vi "Central_Controller_KAFB.vi"() -> ()   [LabVIEW 2019]
uses:
  <vilib>/Modbus/master/Modbus Master.lvclass
  <vilib>/Modbus/master/Create Master Instance (TCP).vi
panel:
  out "ALL Reactive Power":sgl[](array[numeric])
  out "ALL Frequency":sgl[](array[numeric])
  out "ALL Inverter Real Power":sgl[](array[numeric])
  out "ALL Inverter Reactive Power":sgl[](array[numeric])
  out "ALL Generator DC Voltage":sgl[](array[numeric])
  out "ALL Generator DC Current":sgl[](array[numeric])
  out "ALL Solar DC Voltage":sgl[](array[numeric])
  out "ALL Solar DC Current":sgl[](array[numeric])
  in  "DER List":string[](array[string])=["Capstone", "Aquion", "Tesla", "Load Bank", "Motor 1", "Simpliphi 1", "LG Chem", "Outback 1", "Outback 2", "Sunny Island", "ESS", "Fuel Cells", "Sparkplug", "Fronius", "Suny Boy", "Motor 2"]
  out "data":T1
  in  "File Name":string
  out "error out 3":errorcluster
  in  "Folder":path=path "C:/Users/administrator.STONEEDGEPOWER/Desktop/Data"
  out "ALL Status":u16[](array[numeric])
  out "SYS Current Time":dbl format="%.3f"
  out "SYS DER Index":i32
  out "ALL Control Method":string[](array[string])
  out "ALL Logged":bool[](array[boolean])
  out "ALL Through Variable":sgl[](array[numeric])
  out "ALL Across Variable":sgl[](array[numeric])
  out "ALL State of Charge":sgl[](array[numeric])
  out "ALL Real Power":sgl[](array[numeric])
  out "ALL Microgrid Voltage":sgl[](array[numeric])
  in  "Tab Control Main":enum32{"Dashboard", "Comms Control"}(tab)
  out "DER12 Solar Power":sgl format="%#.1f"
  out "DER12 Inverter Power":sgl format="%#.1f"
  out "DER11 Solar Power":sgl format="%#.1f"
  out "DER11 Inverter Power":sgl format="%#.1f"
  out "DER10 Solar Power":sgl format="%#.1f"
  out "DER10 Inverter Power":sgl format="%#.1f"
  out "DER9 Solar Power":sgl format="%#.1f"
  out "DER9 Inverter Power":sgl format="%#.1f"
  out "DER8 Solar Power":sgl format="%#.1f"
  out "DER8 Inverter Power":sgl format="%#.1f"
  out "DER7 Solar Power":sgl format="%#.1f"
  out "DER7 Inverter Power":sgl format="%#.1f"
  out "DER6 Solar Power":sgl format="%#.1f"
  out "DER6 Inverter Power":sgl format="%#.1f"
  out "DER5 Solar Power":sgl format="%#.1f"
  out "DER5 Inverter Power":sgl format="%#.1f"
  out "DER4 Solar Power":sgl format="%#.1f"
  out "DER1 Across Variable":sgl format="%#.1f"
  out "DER0 Across Variable":sgl format="%#.1f"
  out "DER12 Flow":i32(ring)
  out "DER12State of Charge Figure":sgl(slide) scale=0.0..100.0
  out "DER12 State of Charge":sgl format="%#.1f"
  out "DER12 Real Power":sgl format="%.1f"
  in  "DER12 Login Button":bool
  out "DER12 Logged":bool
  out "DER12 DC Voltage":sgl format="%#.1f"
  out "DER12 AC Line-Line Voltage":sgl=209.57935 format="%.1f"
  out "DER12 State":string
  in  "DER12 Control Window Button":bool
  in  "DER12 Detail Window Button":bool
  out "DER11 State of Charge":sgl format="%#.1f"
  out "DER11 Flow":i32(ring)
  in  "DER11 Detail Window Button":bool
  out "DER11 State of Charge Figure":sgl(slide) scale=0.0..100.0
  in  "DER11 Login Button":bool
  out "DER11 Across Variable":sgl format="%#.2f"
  out "DER11 logged":bool
  out "DER11 AC Line-Line Votlage":sgl format="%.1f"
  out "DER11 Real Power":sgl format="%.1f"
  out "DER11 State":string
  in  "DER11 Control Window Button":bool
  out "DER10 Flow":i32(ring)
  out "DER10 State of Charge Figure":sgl(slide) scale=0.0..100.0
  out "DER10 State of Charge":sgl format="%#.1f"
  out "DER10 Real Power":sgl format="%.1f"
  in  "DER10 Login Button":bool
  out "DER10 Logged":bool
  out "DER10 DC Voltage":sgl format="%#.1f"
  out "DER10 AC Line-Line Voltage":sgl=209.57935 format="%.1f"
  out "DER10 State":string
  in  "DER10 Control Window Button":bool
  in  "DER10 Detail Window Button":bool
  out "DER9 State of Charge":sgl format="%#.1f"
  out "DER9 Flow":i32(ring)
  in  "DER9 Detail Window Button":bool
  out "DER9 State of Charge Figure":sgl(slide) scale=0.0..100.0
  in  "DER9 Login Button":bool
  out "DER9 Across Variable":sgl format="%#.2f"
  out "DER9 logged":bool
  out "DER9 AC Line-Line Votlage":sgl format="%.1f"
  out "DER9 Real Power":sgl format="%.1f"
  out "DER9 State":string
  in  "DER9 Control Window Button":bool
  out "DER8 Flow":i32(ring)
  out "DER8 State of Charge Figure":sgl(slide) scale=0.0..100.0
  out "DER8 State of Charge":sgl format="%#.1f"
  out "DER8 Real Power":sgl format="%.1f"
  in  "DER8 Login Button":bool
  out "DER8 Logged":bool
  out "DER8 DC Voltage":sgl format="%#.1f"
  out "DER8 AC Line-Line Voltage":sgl=209.57935 format="%.1f"
  out "DER8 State":string
  in  "DER8 Control Window Button":bool
  in  "DER8 Detail Window Button":bool
  out "DER7 State of Charge":sgl format="%#.1f"
  out "DER5 State of Charge":sgl format="%#.1f"
  out "DER7 Flow":i32(ring)
  in  "DER7 Detail Window Button":bool
  out "DER7 State of Charge Figure":sgl(slide) scale=0.0..100.0
  in  "DER7 Login Button":bool
  out "DER7 Across Variable":sgl format="%#.2f"
  out "DER7 logged":bool
  out "DER7 AC Line-Line Votlage":sgl format="%.1f"
  out "DER7 Real Power":sgl format="%.1f"
  out "DER7 State":string
  in  "DER7 Control Window Button":bool
  out "DER6 Flow":i32(ring)
  out "DER6 State of Charge Figure":sgl(slide) scale=0.0..100.0
  out "DER6 State of Charge":sgl format="%#.1f"
  out "DER6 Real Power":sgl format="%.1f"
  in  "DER6 Login Button":bool
  out "DER6 Logged":bool
  out "DER6 DC Voltage":sgl format="%#.1f"
  out "DER6 AC Line-Line Voltage":sgl=209.57935 format="%.1f"
  out "DER6 State":string
  in  "DER6 Control Window Button":bool
  in  "DER6 Detail Window Button":bool
  out "DER0 State of Charge":sgl format="%.1f"
  out "DER0 State of Charge Figure":sgl(slide) scale=0.0..100.0
  out "DER5 Flow":i32(ring)
  out "DER4 Flow":i32(ring)
  out "DER3 Flow":i32(ring)
  out "DER1 Flow":i32(ring)
  out "DER0 Flow":i32(ring)
  in  "DER2 Detail Window Button":bool
  in  "DER5 Detail Window Button":bool
  out "DER4 State of Charge Figure":sgl(slide) scale=0.0..100.0
  out "DER4 State of Charge":sgl format="%#.1f"
  out "DER4 Real Power":sgl format="%.1f"
  in  "DER4 Login Button":bool
  out "DER4 Logged":bool
  out "DER4 DC Voltage":sgl format="%#.1f"
  out "DER4 AC Line-Line Voltage":sgl=209.57935 format="%.1f"
  out "DER4 State":string
  out "DER5 State of Charge Figure":sgl(slide) scale=0.0..100.0
  in  "DER0 Login Button":bool
  in  "DER2 Login Button":bool
  in  "DER1 Login Button":bool
  out "DER1 Real Power Indicator 1":sgl format="%.1f"
  out "DER1 Reactive Power":sgl format="%#.1f"
  out "DER1 AC Line-Line Voltage":sgl format="%.1f"
  out "DER0 Real Power":sgl format="%#.1f"
  out "DER0 AC Line-Line Voltage":sgl format="%#.1f"
  out "DER2 AC Line-Line Voltage":sgl format="%.1f"
  out "DER2 Real Power":sgl format="%.1f"
  out "DER0 Logged":bool
  out "DER1 Logged":bool
  out "DER2 Logged":bool
  in  "DER3 Login Button":bool
  out "DER3 Logged":bool
  out "DER3 Real Power":sgl format="%#.1f"
  out "DER3 AC Line-Line Votlage":sgl format="%#.1f"
  in  "DER5 Login Button":bool
  out "DER5 Across Variable":sgl format="%#.2f"
  out "DER5 logged":bool
  out "DER5 AC Line-Line Votlage":sgl format="%.1f"
  out "DER5 Real Power":sgl format="%.1f"
  out "DER0 State":string
  out "DER1 State":string
  out "DER2 State":string
  out "DER3 State":string
  out "DER5 State":string
  in  "DER0 Control Window Button":bool
  in  "DER0 Detail Window Button":bool
  in  "DER1 Detail Window Button":bool
  in  "DER1 Control Window Button":bool
  in  "DER2 Control Window Button":bool
  in  "DER3 Control Window Button":bool
  in  "DER5 Control Window Button":bool
  in  "DER4 Control Window Button":bool
  in  "DER4 Detail Window Button":bool
  out "DER2 Control Mode":string="Slave Mode Droops"
  out "DER1 Control Mode":string="Slave Mode Droops"
  out "DER2 Flow":i32(ring)
  out "DER0 Control Mode":string="Slave Mode Droops"
  out "DER1 Real Power Indicator 2":sgl format="%.1f"
  in  "DER3 Detail Window Button":bool
  out "DER1 Frequency":sgl format="%#.1f"
  out "DER4 Inverter Power":sgl format="%#.1f"
  in  "Container":enum32{"Page 1"}(tab)
  in  "DER Type":string[](array[string])=["Central", "Central", "Central", "Central", "Nanogrid", "Nanogrid", "Nanogrid", "Nanogrid", "Nanogrid", "Nanogrid", "Nanogrid", "Nanogrid", "Nanogrid", "DER13", "DER14", "DER15"]
  out "ALL Error Indicator":bool[](array[boolean])
  out "ALL DER Current Error":errorcluster[](array[cluster])
  out "ALL DER Final Error":errorcluster[](array[cluster])
  in  "IP Address List":string[](array[string])=["10.1.32.65", "10.1.32.32", "10.1.32.95", "10.1.32.97", "10.1.32.45", "10.1.32.67", "10.1.32.70", "10.1.32.100", "10.1.32.69", "10.1.32.38", "10.1.32.43", "10.1.32.75", "10.1.32.74", "10.0.1.192", "10.0.1.207", "10.0.1.196"]
  in  "DER Label Name":string[](array[string])=["DER0", "DER1", "DER2", "DER3", "DER4", "DER5", "DER6", "DER7", "DER8", "DER9", "DER10", "DER11", "DER12", "DER13", "DER14", "DER15"]
  out "SYS Iteration":i32
  in  "stop":bool
  out "SYS Status":string="Reading"
  out "SYS Case":i32
  in  "Read Array":bool[](array[boolean])=[TRUE, TRUE, TRUE, TRUE, TRUE, TRUE, TRUE, TRUE, TRUE, TRUE, TRUE, FALSE, TRUE]
  # "DER0: Heila XX, Sinamics, 10.0.8.XX\nDER1: Heila XX, Socomec, 10.0.8.XX\nDER2: Heila XX, Alencon, 10.0.8.XX\nDER3: Heila XX, Polar Power, 10.0.8.XX\nDER4: Heila XX, Nanogrid 1 \nDER5: Heila XX, Nanogrid 2\nDER6: Heila XX, Nanogrid 3\nDER7: Heila XX, Nanogrid 4 \nDER8: Heila XX, Nanogrid 5\nDER9: Heila XX, Nanogrid 6\nDER10: Heila XX, Nanogrid 7 \nDER11: Heila XX, Nanogrid 8\nDER12: Heila XX, Nanogrid 9"
  # "Nanogrid 5"
  # "Nanogrid 7"
  # "Nanogrid 3"
  # "Nanogrid 1"
  # "Nanogrid 9"
  # "House"
  # "DETL"
  # "House"
  # "House"
  # "House"
  # "Battery"
  # "Generators"
  # "Status:"
  # "Status:"
  # "Status:"
  # "Status:"
  # "Status:"
  # "Sinamics + Energport"
  # "EPIC + Polar Power"
  # "V"
  # "V"
  # "V"
  # "V"
  # "V"
  # "Status:"
  # "Status:"
  # "Mode:"
  # "KAFB Microgrid in Real Time"
  # "V"
  # "SoC"
  # "%"
  # "SoC"
  # "%"
  # "SoC"
  # "%"
  # "SoC"
  # "%"
  # "SoC"
  # "%"
  # "Load:"
  # "Load:"
  # "Load:"
  # "Load:"
  # "Load:"
  # "Solar:"
  # "Solar:"
  # "Solar:"
  # "Solar:"
  # "Solar:"
  # "SoC"
  # "%"
  # "Inverter"
  # "Utility Grid"
  # "kW"
  # "kW"
  # "kW"
  # "kW"
  # "kW"
  # "kW"
  # "kW"
  # "kW"
  # "Socomec"
  # "V"
  # "V"
  # "V"
  # "V"
  # "V"
  # "V"
  # "V"
  # "V"
  # "Status:"
  # "Mode:"
  # "V ="
  # "V"
  # "f ="
  # "Hz"
  # "P ="
  # "kW"
  # "kW"
  # "kW"
  # "kW"
  # "kW"
  # "kW"
  # "kVAr"
  # "Q ="
  # "V"
  # "V"
  # "V"
  # "V"
  # "V"
  # "Solar"
  # "Nanogrid 8"
  # "Nanogrid 6"
  # "Nanogrid 4"
  # "Nanogrid 2"
  # "Laundry"
  # "House"
  # "House"
  # "PV + Alencon"
  # "House"
  # "Status:"
  # "Status:"
  # "Status:"
  # "Status:"
  # "Status:"
  # "Mode:"
  # "V"
  # "V"
  # "V"
  # "V"
  # "SoC"
  # "%"
  # "SoC"
  # "%"
  # "SoC"
  # "%"
  # "SoC"
  # "%"
  # "Load:"
  # "Load:"
  # "Load:"
  # "Load:"
  # "Solar:"
  # "Solar:"
  # "Solar:"
  # "Solar:"
  # "Program"
  # "Controllable DERs"
  # "DER0: Heila XX, Sinamics, 10.1.32.65\nDER1: Heila XX, Socomec, 10.1.32.32\nDER2: Heila XX, Alencon, 10.1.32.95\nDER3: Heila XX, Polar Power, 10.1.32.97\nDER4: Heila XX, Nanogrid 1, 10.1.32.45 \nDER5: Heila XX, Nanogrid 2, 10.1.32.67\nDER6: Heila XX, Nanogrid 3, 10.1.32.70\nDER7: Heila XX, Nanogrid 4, 10.1.32.100\nDER8: Heila XX, Nanogrid 5, 10.1.32.68\nDER9: Heila XX, Nanogrid 6, 10.1.32.38\nDER10: Heila XX, Nanogrid 7, 10.1.32.43\nDER11: Heila XX, Nanogrid 8\nDER12: Heila XX, Nanogrid 9"
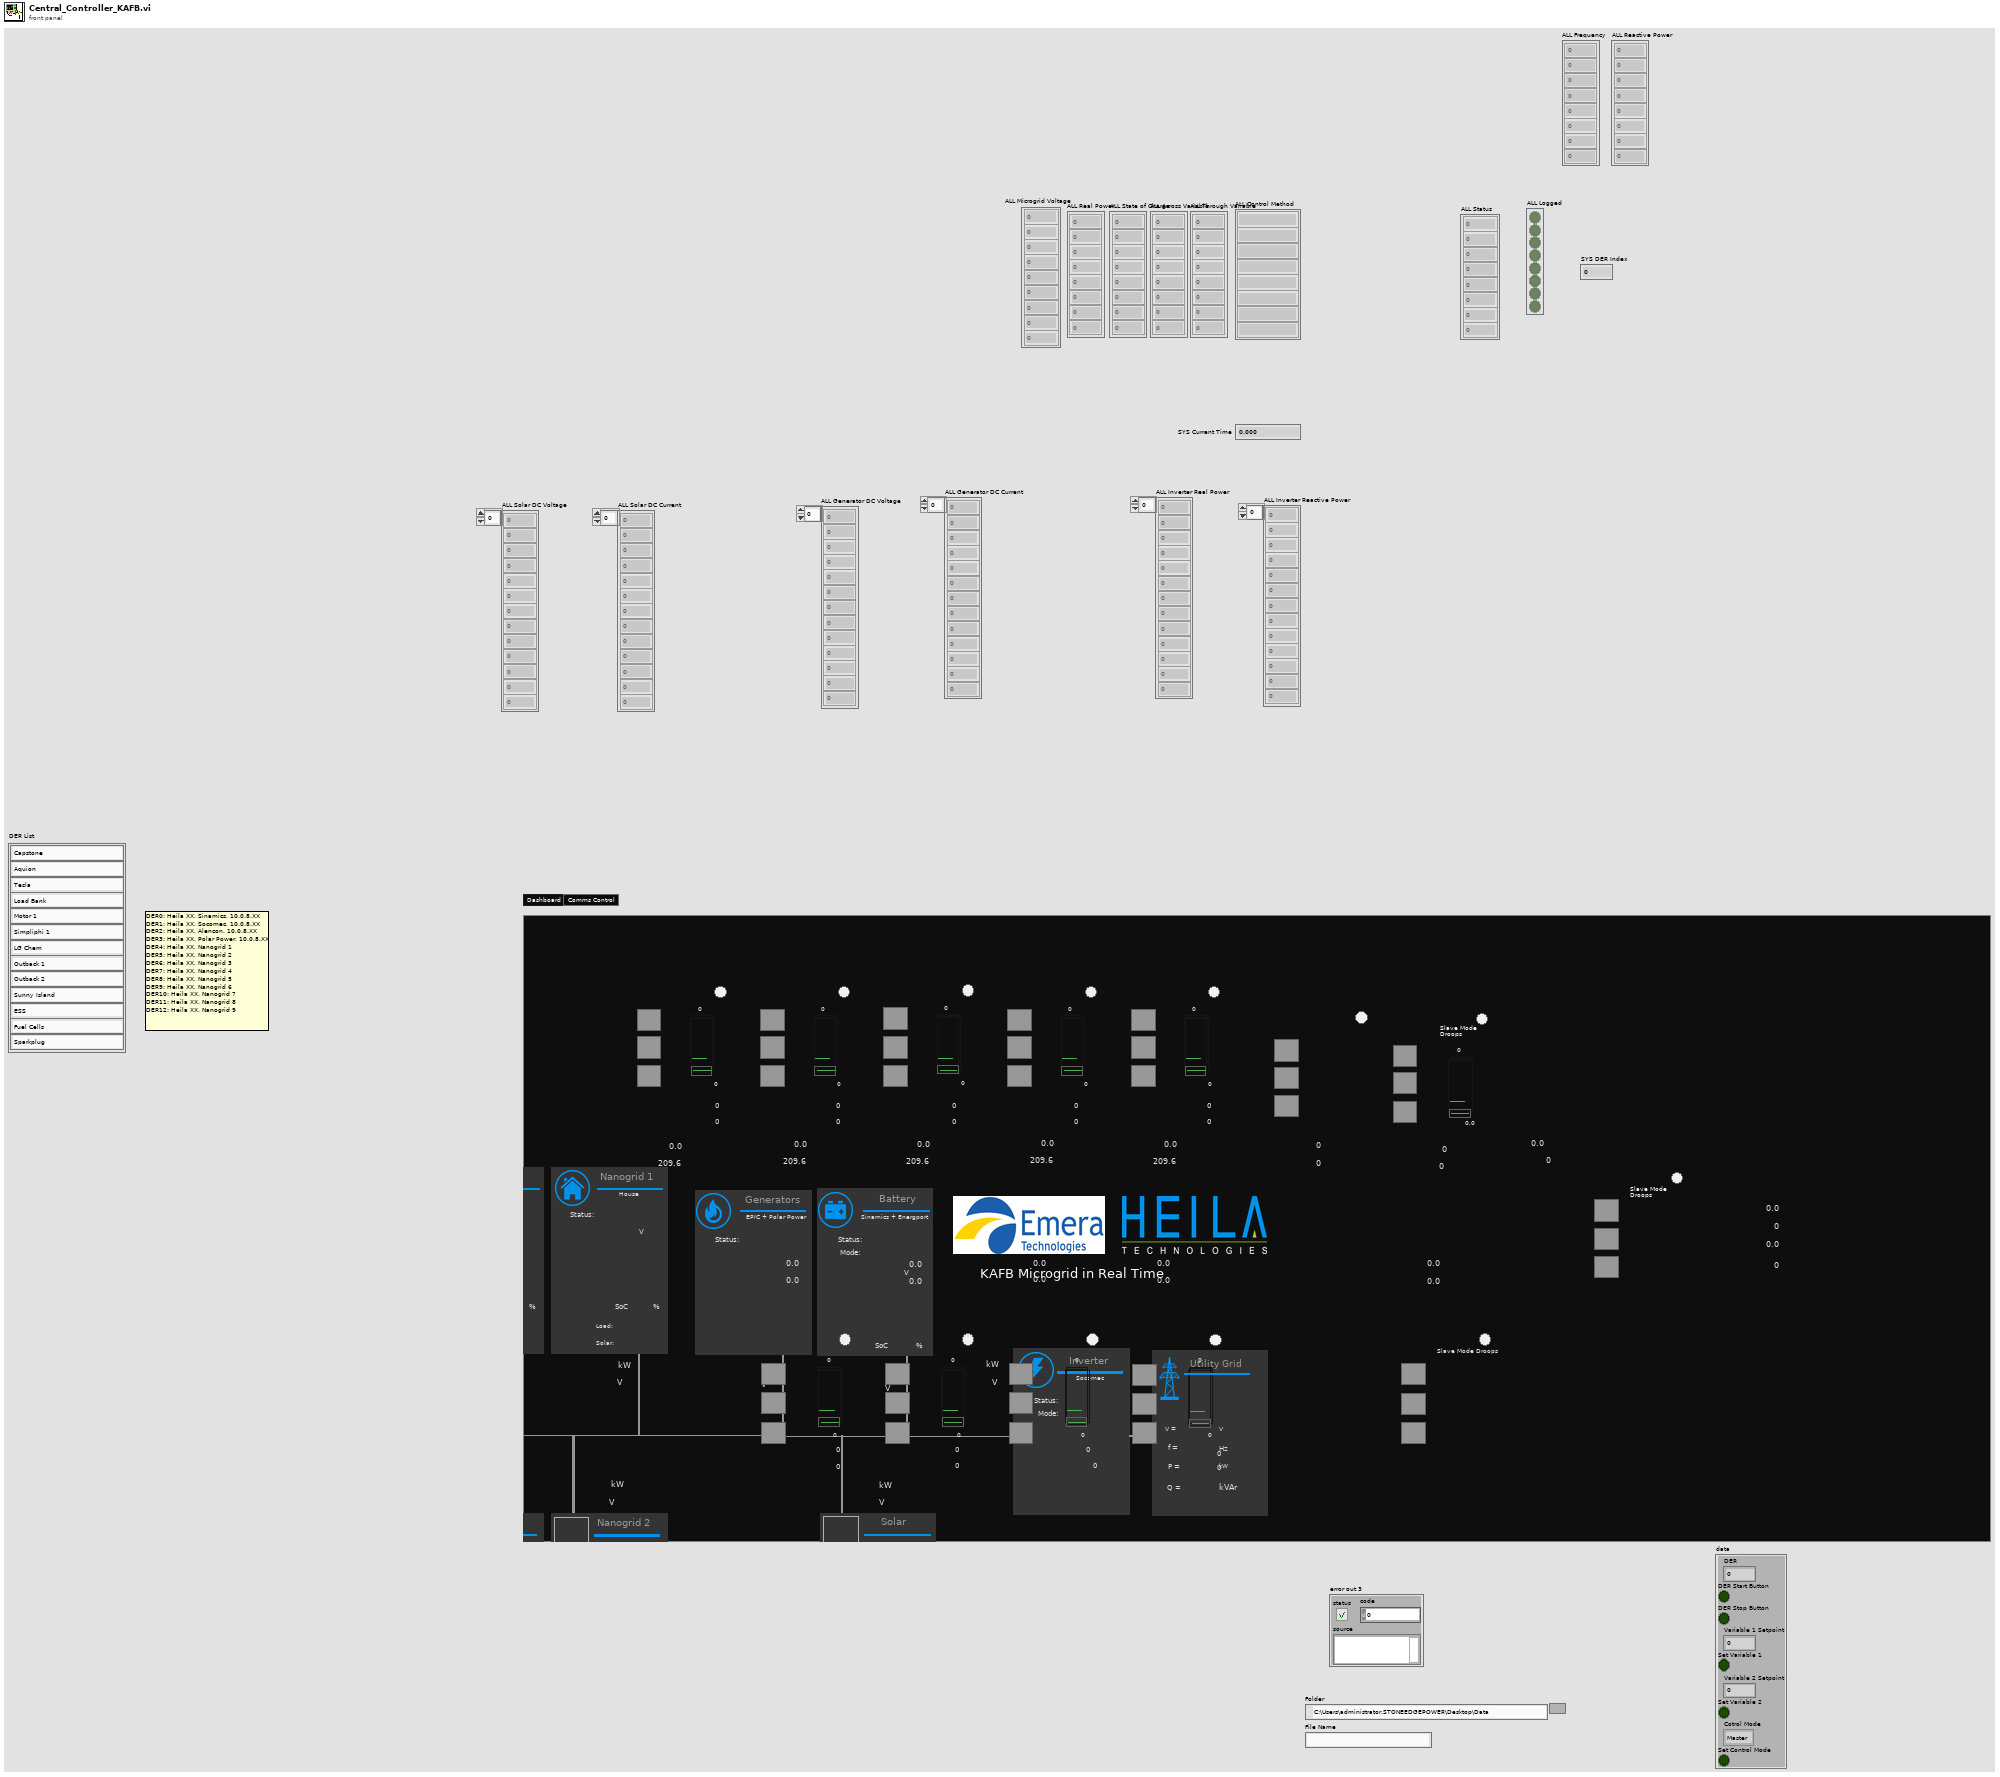
[diagram p1: front panel]
types:
  T1 = cluster{"DER":i32, "DER Start Button":bool, "DER Stop Button":bool, "Variable 1 Setpoint":sgl, "Set Variable 1":bool, "Variable 2 Setpoint":sgl, "Set Variable 2":bool, "Cotrol Mode":enum16{"Master", "Slave"}, "Set Control Mode":bool}
  T2 = enum16{"open", "replace", "create", "open or create", "replace or create", "replace or create with confirmation"}
  T3 = cluster{"Modbus master out":refnum<class "Modbus Master.lvclass">, "error out":errorcluster}[]
  T4 = enum32{"Invalid", "Standard", "Closed", "Hidden", "Minimized", "Maximized"}
  T5 = cluster{"Modbus master out":refnum<class "Modbus Master.lvclass">, "error out":errorcluster}
  T6 = enum32{"Bad", "Idle", "Run top level", "Running"}
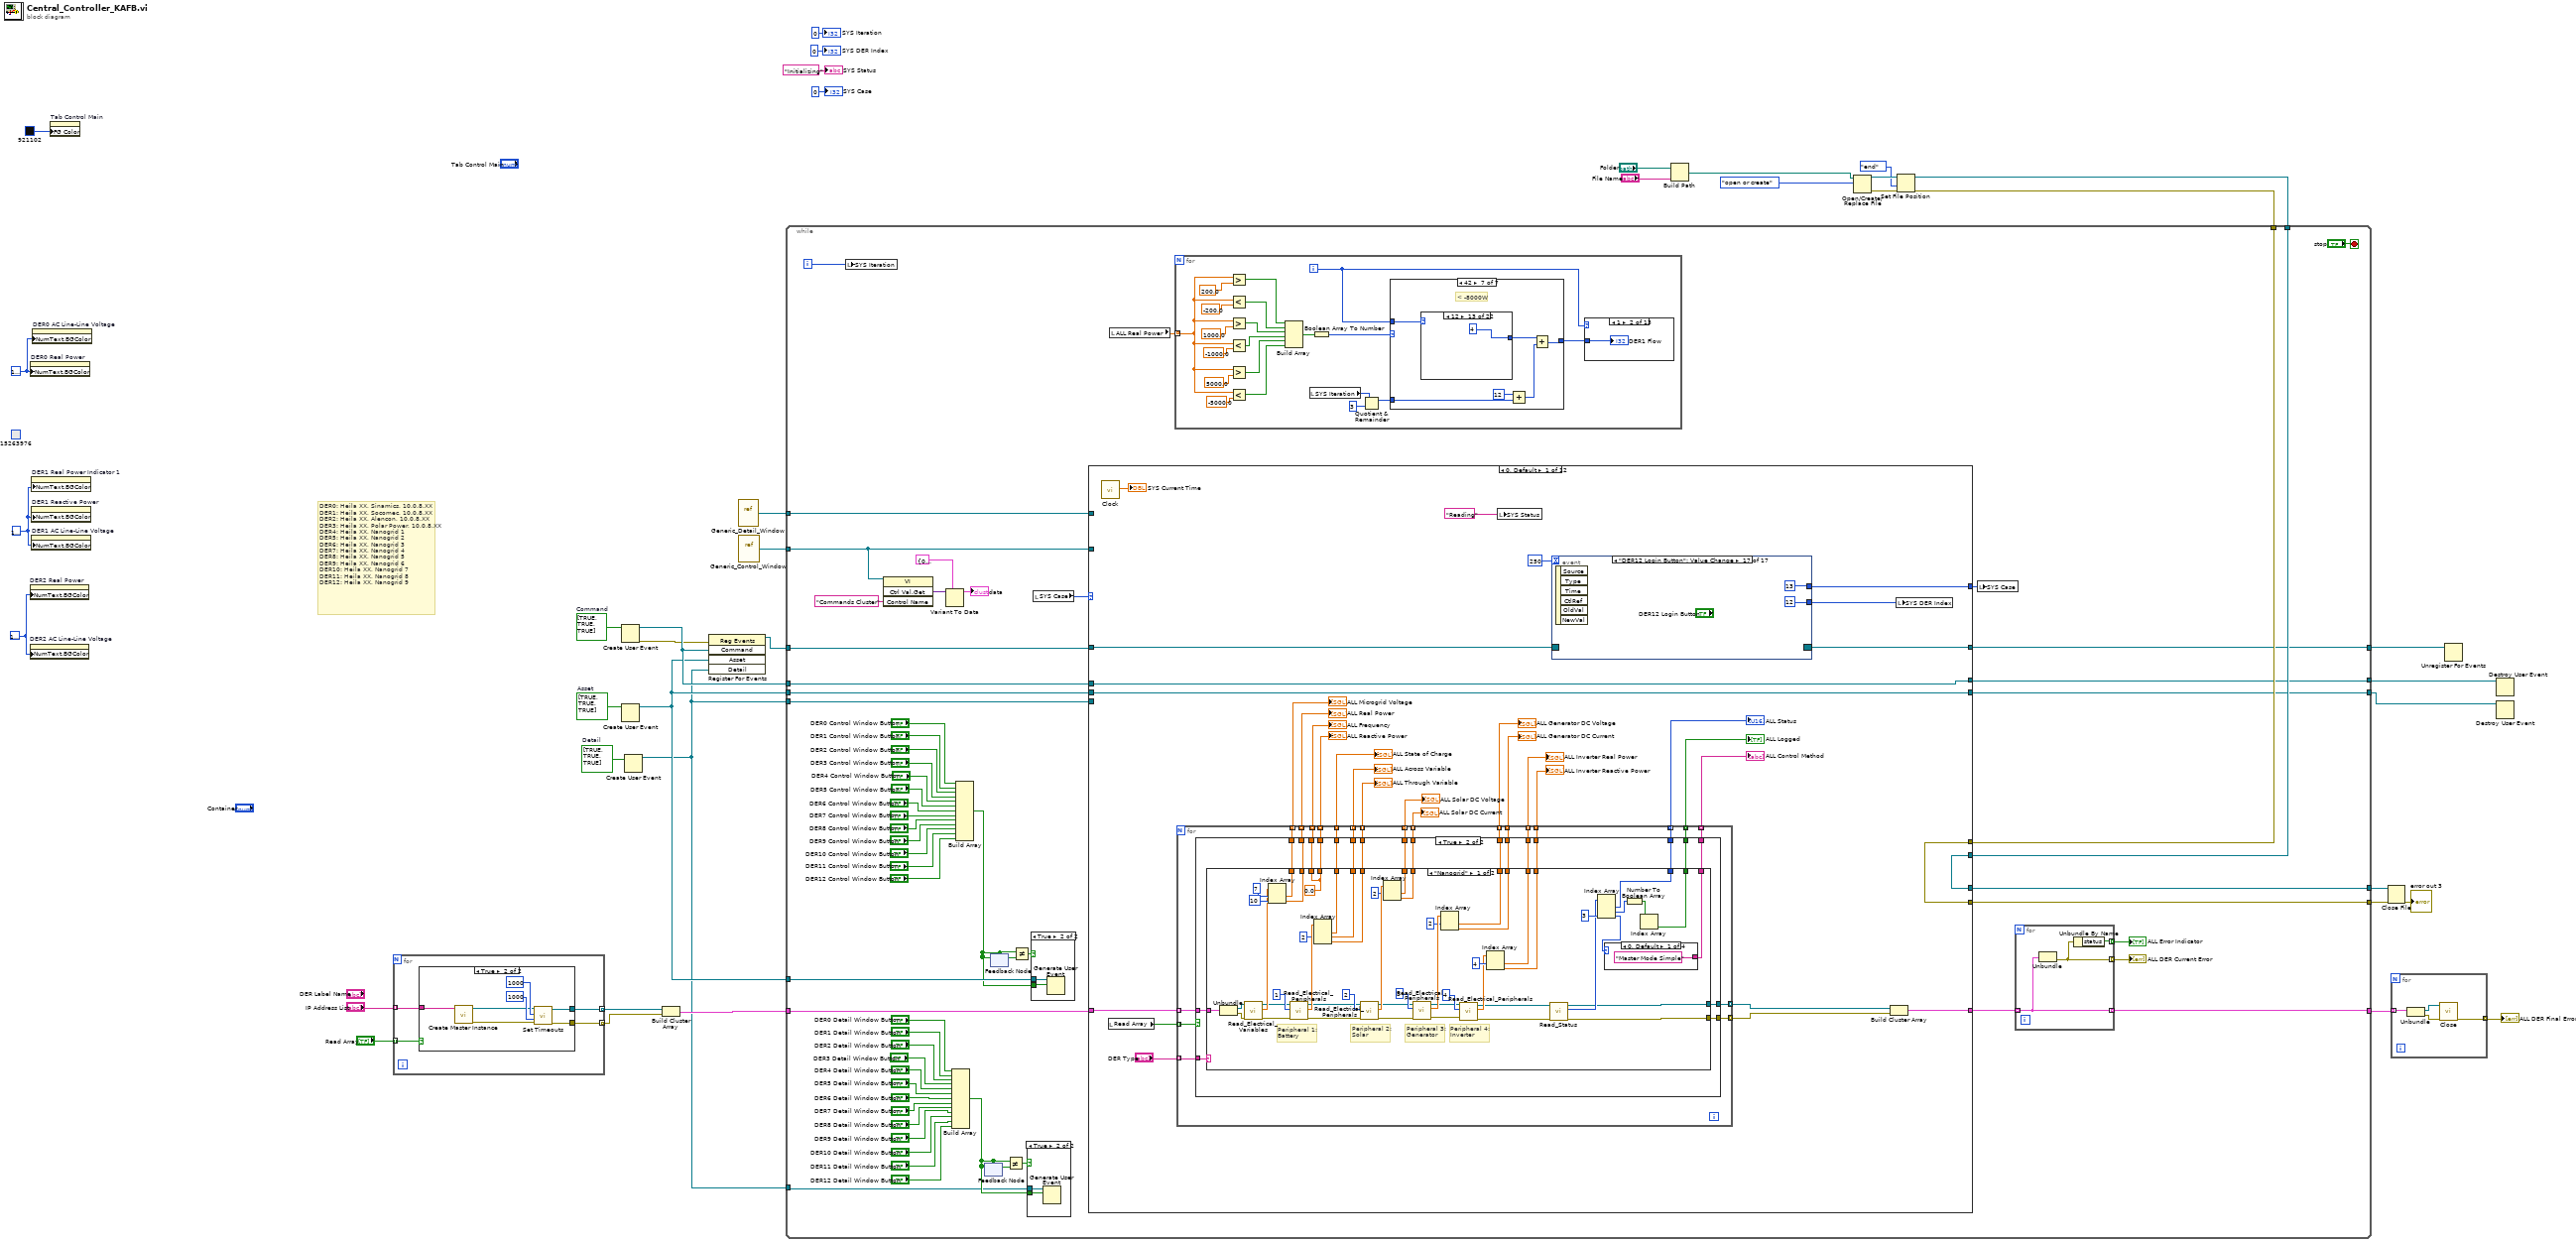
[diagram p0: block diagram]
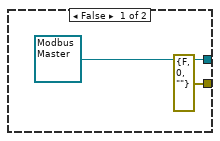
[diagram p2: hidden frame]
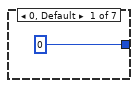
[diagram p5: hidden frame]
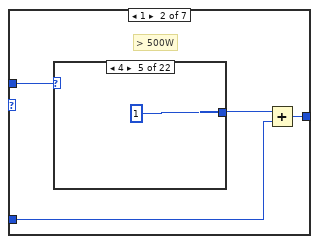
[diagram p6: hidden frame]
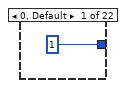
[diagram p7: hidden frame]
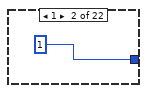
[diagram p8: hidden frame]
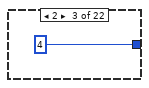
[diagram p9: hidden frame]
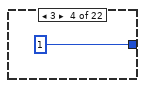
[diagram p10: hidden frame]
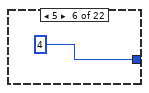
[diagram p11: hidden frame]
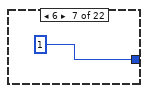
[diagram p12: hidden frame]
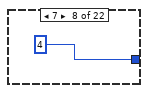
[diagram p13: hidden frame]
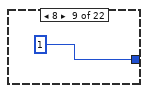
[diagram p14: hidden frame]
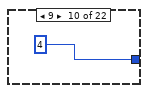
[diagram p15: hidden frame]
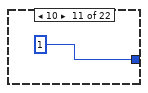
[diagram p16: hidden frame]
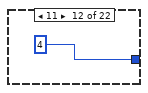
[diagram p17: hidden frame]
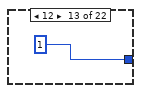
[diagram p18: hidden frame]
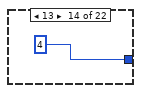
[diagram p19: hidden frame]
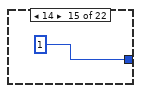
[diagram p20: hidden frame]
diagram:
  w4 = bool[] [TRUE, TRUE, TRUE]  # Detail
  w10 = bool[] [TRUE, TRUE, TRUE]  # Asset
  w13 = bool[] [TRUE, TRUE, TRUE]  # Command
  w36 = u32 16777216
  w37 = u32 16777216
  w38 = u32 16777216
  (unwired) u32 15263976
  # "DER0: Heila XX, Sinamics, 10.0.8.XX\nDER1: Heila XX, Socomec, 10.0.8.XX\nDER2: Heila XX, Alencon, 10.0.8.XX\nDER3: Heila XX, Polar Power, 10.0.8.XX\nDER4: Heila XX, Nanogrid 1 \nDER5: Heila XX, Nanogrid 2\nDER6: Heila XX, Nanogrid 3\nDER7: Heila XX, Nanogrid 4 \nDER8: Heila XX, Nanogrid 5\nDER9: Heila XX, Nanogrid 6\nDER10: Heila XX, Nanogrid 7 \nDER11: Heila XX, Nanogrid 8\nDER12: Heila XX, Nanogrid 9"
  n1 = property on="DER2 Real Power" class="DigNum (strict)"("NumText.BGColor"=w36) -> ()  [unwired: 2 in, 2 out]
  n2 = property on="DER2 AC Line-Line Voltage" class="DigNum (strict)"("NumText.BGColor"=w36) -> ()  [unwired: 2 in, 2 out]
  n3 = property on="DER0 Real Power" class="DigNum (strict)"("NumText.BGColor"=w38) -> ()  [unwired: 2 in, 2 out]
  n4 = property on="DER1 Real Power Indicator 1" class="DigNum (strict)"("NumText.BGColor"=w37) -> ()  [unwired: 2 in, 2 out]
  n5 = property on="DER1 Reactive Power" class="DigNum (strict)"("NumText.BGColor"=w37) -> ()  [unwired: 2 in, 2 out]
  n6 = property on="DER1 AC Line-Line Voltage" class="DigNum (strict)"("NumText.BGColor"=w37) -> ()  [unwired: 2 in, 2 out]
  n7 = property on="DER0 AC Line-Line Voltage" class="DigNum (strict)"("NumText.BGColor"=w38) -> ()  [unwired: 2 in, 2 out]
  n8 = property on="Tab Control Main" class="TabCtl (strict)"("FG Color"=u32 921102) -> ()  [unwired: 2 in, 2 out]
  n9 = for {
    tunnel: "IP Address List" -> [w44] mode=indexing
    tunnel: [w43] -> w35 mode=indexing
    tunnel: [w42] -> w34 mode=indexing
    tunnel: "Read Array" -> [w41] mode=indexing
    n10 = case shown="True" w41 {
      tunnel: w44 -> [_ w53]
      tunnel: [refnum<class "Modbus Master.lvclass"> refnum ("Modbus master out") w50] -> w43
      tunnel: [errorcluster {"status"=FALSE, "code"=0, "source"=""} ("error out") w49] -> w42
      frame False {
      }
      frame True {
        n11 = call-poly <vilib>:"Create Master Instance.vi"("address"=w53) -> ("error out"=w47:errorcluster, "TCP master instance"=w48:refnum<class "Modbus Master.lvclass">)  [unwired: 9 in]
        n12 = call <vilib>:"Set Timeouts.vi"("error in (no error)"=w47, "write operation timeout (ms)"=1000 ("Write Timeout"), "read operation timeout (ms)"=1000 ("Read Timeout"), "Modbus master in"=w48) -> ("error out"=w49:errorcluster, "Modbus master out"=w50:refnum<class "Modbus Master.lvclass">)  [unwired: 6 in]
      }
    }
  }
  n13 = Create User Event(user event datatype=w13) -> (user event=w11:refnum<user-event>, error out=w7:errorcluster)  [unwired: 1 in]
  n14 = Create User Event(user event datatype=w10) -> (user event=w6:refnum<user-event>)  [unwired: 1 in, 1 out]
  n15 = Create User Event(user event datatype=w4) -> (user event=w2:refnum<user-event>)  [unwired: 1 in, 1 out]
  n16 = Build Cluster Array(w35, w34) -> (w33:T3)
  n17 = register-events(error in=w7, w11, w6, w2) -> (reference out=w12:refnum<event-registration>)  [unwired: 1 in, 1 out]
  n18 = vi-ref "Generic_Detail_Window.vi"() -> (w3:refnum<vi>)
  n19 = vi-ref "Generic_Control_Window.vi"() -> (w14:refnum<vi>)
  n20 = Build Path(base path="Folder", name or relative path="File Name") -> (appended path=w15:path)
  n21 = Open/Create/Replace File(file path (use dialog)=w15, operation (0:open)=T2."open or create") -> (refnum out=w25:refnum<file>, error out=w24:errorcluster)  [unwired: 4 in, 1 out]
  n22 = Set File Position(refnum=w25, from (0:start)=enum16{"start", "end", "current"}."end", error in=w24) -> (refnum out=w19:refnum<file>, error out=w18:errorcluster)  [unwired: 1 in]
  n23 = while {
    tunnel: w33 -> [w112]
    tunnel: [w108] -> w27
    tunnel: [w106] -> w22
    tunnel: [w105] -> w21
    tunnel: w19 -> [w104]
    tunnel: w18 -> [w103]
    tunnel: w14 -> [w83]
    tunnel: w11 -> [w101]
    tunnel: w6 -> [w92]
    tunnel: [w89] -> w8
    tunnel: w6 -> [w88]
    tunnel: [w87] -> w5
    tunnel: w12 -> [w102]
    tunnel: [w90] -> w9
    tunnel: w2 -> [w74]
    tunnel: w3 -> [w73]
    tunnel: w2 -> [w72]
    i -> [w55]
    stop <- "stop" stop-if-true
    n24 = local write "SYS Iteration"(w55) -> ()
    n25 = invoke class="VI" method="Ctrl Val.Get"(reference=w83, "Control Name"="Commands Cluster") -> ("Get Control Value Variant"=w100:variant)  [unwired: 2 in, 3 out]
    n26 = Variant To Data(type=T1 {"DER"=0, "DER Start Button"=FALSE, "DER Stop Button"=FALSE, "Variable 1 Setpoint"=0.0, "Set Variable 1"=FALSE, "Variable 2 Setpoint"=0.0, "Set Variable 2"=FALSE, "Cotrol Mode"=enum."Slave", "Set Control Mode"=FALSE} ("Commands Cluster 2"), Variant=w100) -> (data=→"data":T1)  [unwired: 1 in, 1 out]
    n27 = Build Array("DER0 Detail Window Button", "DER1 Detail Window Button", "DER2 Detail Window Button", "DER3 Detail Window Button", "DER4 Detail Window Button", "DER5 Detail Window Button", "DER6 Detail Window Button", "DER7 Detail Window Button", "DER8 Detail Window Button", "DER9 Detail Window Button", "DER10 Detail Window Button", "DER11 Detail Window Button", "DER12 Detail Window Button") -> (w76:bool[])
    n28 = Build Array("DER0 Control Window Button", "DER1 Control Window Button", "DER2 Control Window Button", "DER3 Control Window Button", "DER4 Control Window Button", "DER5 Control Window Button", "DER6 Control Window Button", "DER7 Control Window Button", "DER8 Control Window Button", "DER9 Control Window Button", "DER10 Control Window Button", "DER11 Control Window Button", "DER12 Control Window Button") -> (w91:bool[])
    n29 = feedback #1(w76) -> (w77:bool[])
    n30 = feedback-in #1(w76) -> ()
    n31 = feedback-in #2(w91) -> ()
    n32 = feedback #2(w91) -> (w93:bool[])
    n33 = Not Equal?(x=w76, y=w77) -> (x != y?=w75:bool)
    n34 = Not Equal?(x=w91, y=w93) -> (x != y?=w86:bool)
    n35 = case shown="True" w75 {
      tunnel: w74 -> [_ w116]
      tunnel: w76 -> [_ w115]
      frame False {
      }
      frame True {
        n36 = Generate User Event(user event=w116, event data cluster=w115) -> ()  [unwired: 2 in, 2 out]
      }
    }
    n37 = case shown="True" w86 {
      tunnel: w92 -> [_ w118]
      tunnel: w91 -> [_ w117]
      frame False {
      }
      frame True {
        n38 = Generate User Event(user event=w118, event data cluster=w117) -> ()  [unwired: 2 in, 2 out]
      }
    }
    n39 = local read "SYS Case"() -> (w113:i32)
    n40 = case shown="0, Default" w113 {
      tunnel: [w351 2 0 0 0 0 0 0 0 0 w877 w907] -> w82
      tunnel: [w346 w568 w742 w747 w761 w778 w811 w824 w842 w861 w881 w909] -> w111
      tunnel: w112 -> [w349 w568 w742 w749 w762 w782 w812 w823 w843 w862 w881 w909]
      tunnel: [w336 _ w739 _ _ _ _ _ _ _ _ _] -> w106
      tunnel: [w337 _ w738 _ _ _ _ _ _ _ _ _] -> w105
      tunnel: w104 -> [w336 _ w737 _ _ _ _ _ _ _ _ _]
      tunnel: w103 -> [w337 _ w736 _ _ _ _ _ _ _ _ _]
      tunnel: w83 -> [_ _ _ _ _ _ _ _ _ _ w878 _]
      tunnel: w102 -> [w335 w559 w732 _ _ _ _ _ _ _ _ _]
      tunnel: [w334 w559 w732 _ _ _ _ _ _ _ _ _] -> w90
      tunnel: w101 -> [w333 _ _ _ _ _ _ _ _ _ w880 _]
      tunnel: [w333 _ _ _ _ _ _ _ _ _ _ _] -> w89
      tunnel: w88 -> [w332 _ _ _ _ _ _ _ _ _ _ _]
      tunnel: [w332 _ _ _ _ _ _ _ _ _ _ _] -> w87
      tunnel: w73 -> [_ _ _ _ _ _ _ _ _ _ _ w906]
      tunnel: w72 -> [_ _ _ _ _ _ _ _ _ _ _ _]
      frame 0, Default {
        n41 = call "Clock.vi"() -> ("SYS Current Time"=→"SYS Current Time":dbl)  [unwired: 11 in]
        n42 = local read "Read Array"() -> (w330:bool[])
        n43 = for {
          tunnel: w349 -> [w373] mode=indexing
          tunnel: [w372] -> w348 mode=indexing
          tunnel: [w371] -> w347 mode=indexing
          tunnel: [w364] -> w345 mode=indexing
          tunnel: [w370] -> w344 mode=indexing
          tunnel: [w367] -> w343 mode=indexing
          tunnel: [w366] -> w342 mode=indexing
          tunnel: [w369] -> w340 mode=indexing
          tunnel: [w368] -> w341 mode=indexing
          tunnel: [w365] -> w338 mode=indexing
          tunnel: w330 -> [w363] mode=indexing
          tunnel: "DER Type" -> [w362] mode=indexing
          tunnel: [w361] -> w328 mode=indexing
          tunnel: [w360] -> w326 mode=indexing
          tunnel: [w359] -> w327 mode=indexing
          tunnel: [w358] -> w325 mode=indexing
          tunnel: [w357] -> w324 mode=indexing
          tunnel: [w356] -> w323 mode=indexing
          tunnel: [w355] -> w322 mode=indexing
          tunnel: [w354] -> w321 mode=indexing
          tunnel: [w353] -> w320 mode=indexing
          n44 = case shown="True" w363 {
            tunnel: w373 -> [w377 w400]
            tunnel: [w376 w399] -> w372
            tunnel: [w375 w398] -> w371
            tunnel: [w374 w391] -> w370
            tunnel: ["OFF" w397] -> w369
            tunnel: [FALSE w396] -> w368
            tunnel: [w374 w390] -> w367
            tunnel: [w374 w389] -> w366
            tunnel: [u16 1 ("register") w395] -> w365
            tunnel: [w374 w392] -> w364
            tunnel: w362 -> [_ w394]
            tunnel: [w374 w393] -> w361
            tunnel: [w374 w388] -> w360
            tunnel: [w374 w387] -> w359
            tunnel: [w374 w386] -> w358
            tunnel: [w374 w385] -> w357
            tunnel: [w374 w384] -> w356
            tunnel: [w374 w383] -> w355
            tunnel: [w374 w382] -> w354
            tunnel: [w374 w381] -> w353
            frame False {
              w374 = sgl 0.0
              n45 = Unbundle(w377) -> ("Modbus master out"=w376:refnum<class "Modbus Master.lvclass">, "error out"=w375:errorcluster)
            }
            frame True {
              n46 = case shown="\"Nanogrid\"" w394 {
                tunnel: w400 -> [w448 w486]
                tunnel: [w436 w483] -> w399
                tunnel: [w435 w482] -> w398
                tunnel: [w433 w475] -> w397
                tunnel: [w434 w473] -> w396
                tunnel: [w432 w472] -> w395
                tunnel: [w431 w468] -> w393
                tunnel: [w430 w466] -> w392
                tunnel: [w427 w458] -> w391
                tunnel: [w426 w464] -> w390
                tunnel: [w425 w462] -> w389
                tunnel: [w419 w455] -> w388
                tunnel: [w418 w455] -> w387
                tunnel: [w407 w455] -> w386
                tunnel: [w406 w455] -> w385
                tunnel: [w405 w455] -> w384
                tunnel: [w404 w455] -> w383
                tunnel: [w403 w457] -> w382
                tunnel: [w403 w456] -> w381
                frame "Nanogrid" {
                  w403 = 0.0
                  # "Peripheral 4:\nInverter"
                  # "Peripheral 3:\nGenerator"
                  # "Peripheral 2:\nSolar"
                  # "Peripheral 1:\nBattery"
                  n47 = Unbundle(w448) -> ("Modbus master out"=w450:refnum<class "Modbus Master.lvclass">, "error out"=w449:errorcluster)
                  n48 = call "Read_Electrical_Variables.vi"("error in (no error)"=w449, "Modbus master in"=w450) -> ("error out"=w443:errorcluster, "Variables"=w444:sgl[], "Modbus master out"=w442:refnum<class "Modbus Master.lvclass">)  [unwired: 7 in]
                  n49 = Index Array(array=w444, index #1=7, index #2=10 ("index")) -> (element #1=w431:sgl, element #2=w430:sgl)
                  n50 = call "Read_Electrical_Peripherals.vi"("error in (no error)"=w443, "Peripheral number"=1, "Modbus master in"=w442) -> ("error out"=w420:errorcluster, "Variables"=w429:sgl[], "Modbus master out"=w421:refnum<class "Modbus Master.lvclass">)  [unwired: 6 in]
                  n51 = Index Array(array=w429, index #2=2) -> (element #1=w427:sgl, element #2=w426:sgl, element #3=w425:sgl)  [unwired: 2 in]
                  n52 = call "Read_Electrical_Peripherals.vi"("error in (no error)"=w420, "Peripheral number"=2, "Modbus master in"=w421) -> ("error out"=w412:errorcluster, "Variables"=w423:sgl[], "Modbus master out"=w413:refnum<class "Modbus Master.lvclass">)  [unwired: 6 in]
                  n53 = Index Array(array=w423, index #1=2 ("index")) -> (element #1=w419:sgl, element #2=w418:sgl)  [unwired: 1 in]
                  n54 = call "Read_Electrical_Peripherals.vi"("error in (no error)"=w412, "Peripheral number"=3, "Modbus master in"=w413) -> ("error out"=w410:errorcluster, "Variables"=w416:sgl[], "Modbus master out"=w411:refnum<class "Modbus Master.lvclass">)  [unwired: 6 in]
                  n55 = Index Array(array=w416, index #1=2 ("index")) -> (element #1=w407:sgl, element #2=w406:sgl)  [unwired: 1 in]
                  n56 = call "Read_Electrical_Peripherals.vi"("error in (no error)"=w410, "Peripheral number"=4, "Modbus master in"=w411) -> ("error out"=w401:errorcluster, "Variables"=w408:sgl[], "Modbus master out"=w402:refnum<class "Modbus Master.lvclass">)  [unwired: 6 in]
                  n57 = Index Array(array=w408, index #1=4 ("index")) -> (element #1=w405:sgl, element #2=w404:sgl)  [unwired: 1 in]
                  n58 = call "Read_Status.vi"("error in (no error)"=w401, "Modbus master in"=w402) -> ("error out"=w435:errorcluster, "Variables"=w440:u16[], "Modbus master out"=w436:refnum<class "Modbus Master.lvclass">)  [unwired: 7 in]
                  n59 = Index Array(array=w440, index #3=3) -> (element #1=w432:u16, element #2=w439:u16, element #3=w438:u16)  [unwired: 2 in]
                  n60 = case shown="0, Default" w438 {
                    tunnel: ["Master Mode Simple" "Slave Mode Simple" "Master Mode Droops" "Slave Mode Droops"] -> w433
                    frame 0, Default {
                    }
                    frame 1 {
                    }
                    frame 2 {
                    }
                    frame 3 {
                    }
                  }
                  n61 = Number To Boolean Array(number=w439) -> (Boolean array=w437:bool[])
                  n62 = Index Array(array=w437) -> (element=w434:bool)  [unwired: 1 in]
                }
                frame "Central", Default {
                  w455 = sgl 0.0
                  n63 = Unbundle(w486) -> ("Modbus master out"=w485:refnum<class "Modbus Master.lvclass">, "error out"=w484:errorcluster)
                  n64 = call "Read_Electrical_Variables.vi"("error in (no error)"=w484, "Modbus master in"=w485) -> ("error out"=w470:errorcluster, "Variables"=w480:sgl[], "Modbus master out"=w471:refnum<class "Modbus Master.lvclass">)  [unwired: 7 in]
                  n65 = Index Array(array=w480, index #1=7, index #2=10 ("index"), index #6=17 ("index")) -> (element #1=w468:sgl, element #2=w466:sgl, element #3=w457:sgl, element #5=w456:sgl, element #6=w458:sgl)  [unwired: 3 in, 1 out]
                  n66 = call "Read_Electrical_Peripherals.vi"("error in (no error)"=w470, "Peripheral number"=1, "Modbus master in"=w471) -> ("error out"=w460:errorcluster, "Variables"=w465:sgl[], "Modbus master out"=w461:refnum<class "Modbus Master.lvclass">)  [unwired: 6 in]
                  n67 = Index Array(array=w465, index #1=2) -> (element #1=w464:sgl, element #2=w462:sgl)  [unwired: 1 in]
                  n68 = call "Read_Status.vi"("error in (no error)"=w460, "Modbus master in"=w461) -> ("error out"=w482:errorcluster, "Variables"=w478:u16[], "Modbus master out"=w483:refnum<class "Modbus Master.lvclass">)  [unwired: 7 in]
                  n69 = Index Array(array=w478, index #3=3) -> (element #1=w472:u16, element #2=w477:u16, element #3=w476:u16)  [unwired: 2 in]
                  n70 = case shown="0, Default" w476 {
                    tunnel: ["Master Mode Simple" "Slave Mode Simple" "Master Mode Droops" "Slave Mode Droops"] -> w475
                    frame 0, Default {
                    }
                    frame 1 {
                    }
                    frame 2 {
                    }
                    frame 3 {
                    }
                  }
                  n71 = Number To Boolean Array(number=w477) -> (Boolean array=w474:bool[])
                  n72 = Index Array(array=w474) -> (element=w473:bool)  [unwired: 1 in]
                }
              }
            }
          }
        }
        "ALL Microgrid Voltage" <- w328
        "ALL Real Power" <- w345
        "ALL State of Charge" <- w344
        "ALL Across Variable" <- w343
        "ALL Through Variable" <- w342
        "ALL Logged" <- w341
        "ALL Control Method" <- w340
        "ALL Status" <- w338
        "ALL Solar DC Current" <- w327
        "ALL Solar DC Voltage" <- w326
        "ALL Generator DC Current" <- w324
        "ALL Generator DC Voltage" <- w325
        "ALL Inverter Reactive Power" <- w322
        "ALL Inverter Real Power" <- w323
        "ALL Frequency" <- w321
        "ALL Reactive Power" <- w320
        n73 = local write "SYS Status"("Reading") -> ()
        n74 = event shown="[16] \"DER12 Login Button\": Value Change" {
          selector: w335 -> [w491 _ _ _ w527 _ _ _ _ _ _ _ _ _ _ _ _]
          dyn-events: [w491 _ _ _ w527 _ _ _ _ _ _ _ _ _ _ _ _] -> w334
          timeout: 250 -> [_ _ _ _ _ _ _ _ _ _ _ _ _ _ _ _ _]
          tunnel: [1 w496 w507 w517 13 13 13 13 13 13 13 13 13 13 13 13 13] -> w351
          tunnel: [0 w495 w505 w516 0 1 2 3 4 5 6 7 8 9 10 11 12] -> w339
          event Timeout {
            n75 = event-data() -> ()  [unwired: 1 in, 1 out]
          }
          event User Event {
            n76 = event-data() -> ("Asset"=w500:bool[])  [unwired: 1 in]
            n77 = Search 1D Array(1D array=w500, element=TRUE) -> (index of element=w494:i32)  [unwired: 1 in]
            n78 = Equal?(x=w494, y=-1) -> (x = y?=w497:bool)
            n79 = case shown="False" w497 {
              tunnel: [1000 0] -> w496
              tunnel: [w501 0 ("index of element")] -> w495
              tunnel: w494 -> [w501 _]
              frame False {
              }
              frame True {
              }
            }
          }
          event User Event {
            n80 = event-data() -> ("Command"=w508:bool[])  [unwired: 1 in]
            n81 = Boolean Array To Number(Boolean array=w508) -> (number=w509:u32)
            n82 = case shown="0, Default" w509 {
              tunnel: [0 11 12 14 15 500] -> w507
              frame 0, Default {
              }
              frame 1 {
              }
              frame 2 {
              }
              frame 4 {
              }
              frame 8 {
              }
              frame 16 {
              }
            }
            n83 = local read "data"() -> (w506:T1)
            n84 = Unbundle By Name(w506) -> ("DER"=w505:i32)
          }
          event User Event {
            n85 = event-data() -> ("Detail"=w521:bool[])  [unwired: 1 in]
            n86 = Search 1D Array(1D array=w521, element=TRUE) -> (index of element=w518:i32)  [unwired: 1 in]
            n87 = Equal?(x=w518, y=-1) -> (x = y?=w519:bool)
            n88 = case shown="False" w519 {
              tunnel: [1001 0] -> w517
              tunnel: [w523 0 ("index of element")] -> w516
              tunnel: w518 -> [w523 _]
              frame False {
              }
              frame True {
              }
            }
          }
          event "DER0 Login Button": Value Change {
            n89 = event-data() -> ()  [unwired: 1 in, 1 out]
          }
          event "DER1 Login Button": Value Change {
            n90 = event-data() -> ()  [unwired: 1 in, 1 out]
          }
          event "DER2 Login Button": Value Change {
            n91 = event-data() -> ()  [unwired: 1 in, 1 out]
          }
          event "DER3 Login Button": Value Change {
            n92 = event-data() -> ()  [unwired: 1 in, 1 out]
          }
          event "DER4 Login Button": Value Change {
            n93 = event-data() -> ()  [unwired: 1 in, 6 out]
          }
          event "DER5 Login Button": Value Change {
            n94 = event-data() -> ()  [unwired: 1 in, 1 out]
          }
          event "DER6 Login Button": Value Change {
            n95 = event-data() -> ()  [unwired: 1 in, 6 out]
          }
          event "DER7 Login Button": Value Change {
            n96 = event-data() -> ()  [unwired: 1 in, 6 out]
          }
          event "DER8 Login Button": Value Change {
            n97 = event-data() -> ()  [unwired: 1 in, 6 out]
          }
          event "DER9 Login Button": Value Change {
            n98 = event-data() -> ()  [unwired: 1 in, 6 out]
          }
          event "DER10 Login Button": Value Change {
            n99 = event-data() -> ()  [unwired: 1 in, 6 out]
          }
          event "DER11 Login Button": Value Change {
            n100 = event-data() -> ()  [unwired: 1 in, 6 out]
          }
          event "DER12 Login Button": Value Change {
            n101 = event-data() -> ()  [unwired: 1 in, 6 out]
          }
        }
        n102 = Build Cluster Array(w348, w347) -> (w346:T3)
        n103 = local write "SYS DER Index"(w339) -> ()
      }
      frame 1 {
        # "DER0: Heila XX, Sinamics, 10.0.8.XX\nDER1: Heila XX, Socomec, 10.0.8.XX\nDER2: Heila XX, Alencon, 10.0.8.XX\nDER3: Heila XX, Polar Power, 10.0.8.XX\nDER4: Heila XX, Nanogrid 1 \nDER5: Heila XX, Nanogrid 2\nDER6: Heila XX, Nanogrid 3\nDER7: Heila XX, Nanogrid 4 \nDER8: Heila XX, Nanogrid 5\nDER9: Heila XX, Nanogrid 6\nDER10: Heila XX, Nanogrid 7 \nDER11: Heila XX, Nanogrid 8\nDER12: Heila XX, Nanogrid 9"
        n104 = local read "ALL Solar DC Current"() -> (w555:sgl[])
        n105 = local read "ALL Generator DC Current"() -> (w554:sgl[])
        n106 = local read "ALL Inverter Real Power"() -> (w556:sgl[])
        n107 = local read "ALL Microgrid Voltage"() -> (w567:sgl[])
        n108 = local read "ALL Real Power"() -> (w566:sgl[])
        n109 = local read "ALL Frequency"() -> (w557:sgl[])
        n110 = local read "ALL Reactive Power"() -> (w558:sgl[])
        n111 = local read "ALL State of Charge"() -> (w565:sgl[])
        n112 = local read "ALL Across Variable"() -> (w561:sgl[])
        n113 = local read "ALL Through Variable"() -> (w560:sgl[])
        n114 = local read "ALL Status"() -> (w564:u16[])
        n115 = local read "ALL Logged"() -> (w563:bool[])
        n116 = local read "ALL Control Method"() -> (w562:string[])
        n117 = for {
          tunnel: w567 -> [w585] mode=indexing
          tunnel: w566 -> [w584] mode=indexing
          tunnel: w565 -> [w583] mode=indexing
          tunnel: w564 -> [w578] mode=indexing
          tunnel: w563 -> [w582] mode=indexing
          tunnel: w562 -> [w581] mode=indexing
          tunnel: w561 -> [w580] mode=indexing
          tunnel: w560 -> [w579] mode=indexing
          tunnel: w558 -> [w576] mode=indexing
          tunnel: w557 -> [w575] mode=indexing
          tunnel: w556 -> [w574] mode=indexing
          tunnel: w555 -> [w573] mode=indexing
          tunnel: w554 -> [w572] mode=indexing
          i -> [w586]
          n118 = case shown="8" w578 {
            tunnel: ["Operating" "Off" "Sleeping" "Starting" "Stopping" "Busy" "6: N/A" "Fault" "Standby" "Generic Failure"] -> w577
            frame 0, Default {
            }
            frame 1 {
            }
            frame 2 {
            }
            frame 3 {
            }
            frame 4 {
            }
            frame 5 {
            }
            frame 6 {
            }
            frame 7 {
            }
            frame 8 {
            }
            frame 65535 {
            }
          }
          n119 = case shown="4" w586 {
            tunnel: w585 -> [w598 w610 w618 w625 w635 w646 w657 w668 w679 w690 w701 w715 w726]
            tunnel: w584 -> [w604 w615 w620 w628 w638 w651 w658 w670 w680 w692 w703 w713 w724]
            tunnel: w583 -> [w601 _ _ _ w636 w647 w663 w673 w683 w694 w705 w718 w727]
            tunnel: w582 -> [w605 w617 w623 w626 w640 w652 w661 w672 w685 w696 w707 w717 w728]
            tunnel: w581 -> [w599 w616 w624 _ _ _ _ _ _ _ _ w716 _]
            tunnel: w580 -> [w597 w609 _ _ w633 w644 w656 w667 w678 w689 w700 w711 w722]
            tunnel: w579 -> [_ _ _ _ _ _ _ _ _ _ _ _ _]
            tunnel: w577 -> [w600 w611 w619 w627 w641 w648 w662 w674 w684 w695 w706 _ w729]
            tunnel: w576 -> [_ w607 _ _ _ _ _ _ _ _ _ _ _]
            tunnel: w575 -> [_ w606 _ _ _ _ _ _ _ _ _ _ _]
            tunnel: w574 -> [_ _ _ _ w631 w642 w653 w664 w675 w686 w697 w708 w719]
            tunnel: w573 -> [_ _ _ _ w632 w645 w655 w666 w677 w688 w699 w710 w721]
            tunnel: w572 -> [_ _ _ _ _ _ _ _ _ _ _ _ _]
            frame 0, Default {
              n120 = Divide(x=w604, y=sgl 1000.0) -> (x/y=→"DER0 Real Power":sgl)
              "DER0 AC Line-Line Voltage" <- w598
              "DER0 Logged" <- w605
              "DER0 State" <- w600
              "DER0 State of Charge Figure" <- w601
              "DER0 State of Charge" <- w601
              "DER0 Control Mode" <- w599
              "DER0 Across Variable" <- w597
            }
            frame 1 {
              n121 = Divide(x=w607, y=sgl 1000.0) -> (x/y=→"DER1 Reactive Power":sgl)
              n122 = Divide(x=w615, y=sgl 1000.0) -> (x/y=→"DER1 Real Power Indicator 1" →"DER1 Real Power Indicator 2":sgl)
              "DER1 AC Line-Line Voltage" <- w610
              "DER1 Logged" <- w617
              "DER1 Control Mode" <- w616
              "DER1 State" <- w611
              "DER1 Across Variable" <- w609
              "DER1 Frequency" <- w606
            }
            frame 2 {
              n123 = Divide(x=w620, y=sgl 1000.0) -> (x/y=→"DER2 Real Power":sgl)
              "DER2 Logged" <- w623
              "DER2 Control Mode" <- w624
              "DER2 AC Line-Line Voltage" <- w618
              "DER2 State" <- w619
            }
            frame 3 {
              n124 = Divide(x=w628, y=1000.0) -> (x/y=→"DER3 Real Power":dbl)
              "DER3 Logged" <- w626
              "DER3 State" <- w627
              "DER3 AC Line-Line Votlage" <- w625
            }
            frame 4 {
              n125 = Divide(x=w638, y=sgl 1000.0) -> (x/y=→"DER4 Real Power":sgl)
              n126 = Multiply(x=w633, y=w632) -> (x*y=→"DER4 Solar Power":sgl)
              "DER4 DC Voltage" <- w633
              "DER4 AC Line-Line Voltage" <- w635
              "DER4 State" <- w641
              "DER4 Logged" <- w640
              "DER4 State of Charge" <- w636
              "DER4 State of Charge Figure" <- w636
              "DER4 Inverter Power" <- w631
            }
            frame 5 {
              n127 = Divide(x=w651, y=sgl 1000.0) -> (x/y=→"DER5 Real Power":sgl)
              n128 = Multiply(x=w645, y=w644) -> (x*y=→"DER5 Solar Power":sgl)
              "DER5 Across Variable" <- w644
              "DER5 logged" <- w652
              "DER5 State of Charge Figure" <- w647
              "DER5 AC Line-Line Votlage" <- w646
              "DER5 State" <- w648
              "DER5 State of Charge" <- w647
              "DER5 Inverter Power" <- w642
            }
            frame 6 {
              n129 = Divide(x=w658, y=sgl 1000.0) -> (x/y=→"DER6 Real Power":sgl)
              n130 = Multiply(x=w656, y=w655) -> (x*y=→"DER6 Inverter Power":sgl)
              "DER6 State" <- w662
              "DER6 AC Line-Line Voltage" <- w657
              "DER6 DC Voltage" <- w656
              "DER6 Logged" <- w661
              "DER6 State of Charge" <- w663
              "DER6 State of Charge Figure" <- w663
              "DER6 Solar Power" <- w653
            }
            frame 7 {
              n131 = Divide(x=w670, y=sgl 1000.0) -> (x/y=→"DER7 Real Power":sgl)
              n132 = Multiply(x=w667, y=w666) -> (x*y=→"DER7 Solar Power":sgl)
              "DER7 State of Charge Figure" <- w673
              "DER7 Across Variable" <- w667
              "DER7 State" <- w674
              "DER7 AC Line-Line Votlage" <- w668
              "DER7 State of Charge" <- w673
              "DER7 logged" <- w672
              "DER7 Inverter Power" <- w664
            }
            frame 8 {
              n133 = Multiply(x=w678, y=w677) -> (x*y=→"DER8 Solar Power":sgl)
              n134 = Divide(x=w680, y=sgl 1000.0) -> (x/y=→"DER8 Real Power":sgl)
              "DER8 State" <- w684
              "DER8 AC Line-Line Voltage" <- w679
              "DER8 DC Voltage" <- w678
              "DER8 Logged" <- w685
              "DER8 State of Charge" <- w683
              "DER8 State of Charge Figure" <- w683
              "DER8 Inverter Power" <- w675
            }
            frame 9 {
              n135 = Multiply(x=w689, y=w688) -> (x*y=→"DER9 Solar Power":sgl)
              n136 = Divide(x=w692, y=sgl 1000.0) -> (x/y=→"DER9 Real Power":sgl)
              "DER9 State" <- w695
              "DER9 AC Line-Line Votlage" <- w690
              "DER9 logged" <- w696
              "DER9 Across Variable" <- w689
              "DER9 State of Charge Figure" <- w694
              "DER9 State of Charge" <- w694
              "DER9 Inverter Power" <- w686
            }
            frame 10 {
              n137 = Multiply(x=w700, y=w699) -> (x*y=→"DER10 Solar Power":sgl)
              n138 = Divide(x=w703, y=sgl 1000.0) -> (x/y=→"DER10 Real Power":sgl)
              "DER10 State" <- w706
              "DER10 DC Voltage" <- w700
              "DER10 Logged" <- w707
              "DER10 State of Charge Figure" <- w705
              "DER10 State of Charge" <- w705
              "DER10 AC Line-Line Voltage" <- w701
              "DER10 Inverter Power" <- w697
            }
            frame 11 {
              n139 = Divide(x=w713, y=sgl 1000.0) -> (x/y=→"DER11 Real Power":sgl)
              n140 = Multiply(x=w711, y=w710) -> (x*y=→"DER11 Solar Power":sgl)
              "DER11 AC Line-Line Votlage" <- w715
              "DER11 logged" <- w717
              "DER11 State" <- w716
              "DER11 Across Variable" <- w711
              "DER11 State of Charge" <- w718
              "DER11 State of Charge Figure" <- w718
              "DER11 Inverter Power" <- w708
            }
            frame 12 {
              n141 = Divide(x=w724, y=sgl 1000.0) -> (x/y=→"DER12 Real Power":sgl)
              n142 = Multiply(x=w722, y=w721) -> (x*y=→"DER12 Solar Power":sgl)
              "DER12 State" <- w729
              "DER12 Logged" <- w728
              "DER12 DC Voltage" <- w722
              "DER12 State of Charge" <- w727
              "DER12State of Charge Figure" <- w727
              "DER12 AC Line-Line Voltage" <- w726
              "DER12 Inverter Power" <- w719
            }
          }
        }
        n143 = local write "SYS Status"("Processing" ("Status")) -> ()
        n144 = Wait Until Next ms Multiple(millisecond multiple=u32 250) -> ()  [unwired: 1 out]
      }
      frame 2 {
        n145 = local read "SYS Current Time"() -> (w731:dbl)
        n146 = local write "SYS Status"("Saving" ("Status")) -> ()
        n147 = Build Array(w731) -> (w735:dbl[])
        n148 = Reshape Array(w735, 19 ("dimension size")) -> (w734:dbl[])
        n149 = Array To Spreadsheet String(array=w734, 3:"%f" ("format string")) -> (spreadsheet string=w740:string)  [unwired: 1 in]
        n150 = Write to Text File(file (use dialog)=w737, text=w740, error in=w736) -> (refnum out=w739:refnum<file>, error out=w738:errorcluster)  [unwired: 1 in, 1 out]
        n151 = Wait Until Next ms Multiple(millisecond multiple=u32 250) -> ()  [unwired: 1 out]
      }
      frame 11 {
        n152 = local read "SYS DER Index"() -> (w745:i32)
        n153 = Index Array(array=w749, index=w745) -> (element=w754:T5)
        n154 = Unbundle(w754) -> ("Modbus master out"=w753:refnum<class "Modbus Master.lvclass">, "error out"=w752:errorcluster)
        n155 = local write "SYS Status"("Start" ("Status")) -> ()
        n156 = call-dynamic "Write Single Holding Register.vi"("error in (no error)"=w752, "holding register value"=u16 1, "address"=u16 2032 ("starting address"), "Modbus master in"=w753) -> ("error out"=w750:errorcluster, "Modbus master out"=w751:refnum<class "Modbus Master.lvclass">)  [unwired: 6 in]
        n157 = Bundle("Modbus master out"=w751, "error out"=w750) -> (w748:T5)  [unwired: 1 in]
        n158 = Wait Until Next ms Multiple(millisecond multiple=u32 250) -> ()  [unwired: 1 out]
        n159 = Replace Array Subset(array=w749, new element=w748, index=w745) -> (w747:T3)
      }
      frame 12 {
        n160 = local read "SYS DER Index"() -> (w760:i32)
        n161 = Index Array(array=w762, index=w760) -> (element=w768:T5)
        n162 = Unbundle(w768) -> ("Modbus master out"=w767:refnum<class "Modbus Master.lvclass">, "error out"=w766:errorcluster)
        n163 = local write "SYS Status"("Stop" ("Status")) -> ()
        n164 = call-dynamic "Write Single Holding Register.vi"("error in (no error)"=w766, "holding register value"=u16 0, "address"=u16 2032 ("starting address"), "Modbus master in"=w767) -> ("error out"=w764:errorcluster, "Modbus master out"=w765:refnum<class "Modbus Master.lvclass">)  [unwired: 6 in]
        n165 = Bundle("Modbus master out"=w765, "error out"=w764) -> (w763:T5)  [unwired: 1 in]
        n166 = Replace Array Subset(array=w762, new element=w763, index=w760) -> (w761:T3)
        n167 = Wait Until Next ms Multiple(millisecond multiple=u32 250) -> ()  [unwired: 1 out]
      }
      frame 13 {
        n168 = local read "SYS DER Index"() -> (w773:i32)
        n169 = String To Byte Array(string="HEILA") -> (unsigned byte array=w788:u8[])
        n170 = Index Array(array=w782, index=w773) -> (element=w784:T5)
        n171 = for {
          N: 16 -> [_]
          tunnel: w788 -> [w799]
          tunnel: [w798] -> w776 mode=indexing
          i -> [w794]
          n172 = Multiply(x=w794, y=2) -> (x*y=w795:i32)
          n173 = Increment(x=w795) -> (x+1=w796:i32)
          n174 = Index Array(array=w799, index #1=w795, index #2=w796) -> (element #1=w793:u8, element #2=w791:u8)
          n175 = To Unsigned Byte Integer(number=w793) -> (unsigned 8bit integer=w792:u8)
          n176 = To Unsigned Byte Integer(number=w791) -> (unsigned 8bit integer=w790:u8)
          n177 = Join Numbers(hi=w792, lo=w790) -> ((hi.lo)=w798:u16)
        }
        n178 = Unbundle(w784) -> ("Modbus master out"=w777:refnum<class "Modbus Master.lvclass">, "error out"=w783:errorcluster)
        n179 = call-dynamic "Write Multiple Holding Registers.vi"("error in (no error)"=w783, "holding register values"=w776, "starting address"=u16 2000, "Modbus master in"=w777) -> ("error out"=w780:errorcluster, "Modbus master out"=w781:refnum<class "Modbus Master.lvclass">)  [unwired: 6 in]
        n180 = local write "SYS Status"("Login" ("Status")) -> ()
        n181 = Bundle("Modbus master out"=w781, "error out"=w780) -> (w779:T5)  [unwired: 1 in]
        n182 = Replace Array Subset(array=w782, new element=w779, index=w773) -> (w778:T3)
        n183 = Wait Until Next ms Multiple(millisecond multiple=u32 250) -> ()  [unwired: 1 out]
      }
      frame 14 {
        n184 = local read "SYS DER Index"() -> (w803:i32)
        n185 = Index Array(array=w812, index=w803) -> (element=w813:T5)
        n186 = local read "data"() -> (w800:T1)
        n187 = Unbundle By Name(w800) -> ("Variable 1 Setpoint"=w801:sgl)
        n188 = Type Cast(type=u32 0, x=w801) -> (*(type *) &x=w818:u32)
        n189 = Split Number(x=w818) -> (hi(x)=w816:u16, lo(x)=w815:u16)
        n190 = Unbundle(w813) -> ("Modbus master out"=w810:refnum<class "Modbus Master.lvclass">, "error out"=w809:errorcluster)
        n191 = Build Array(w816, w815) -> (w804:u16[])
        n192 = call-dynamic "Write Multiple Holding Registers.vi"("error in (no error)"=w809, "holding register values"=w804, "starting address"=u16 2036, "Modbus master in"=w810) -> ("error out"=w807:errorcluster, "Modbus master out"=w808:refnum<class "Modbus Master.lvclass">)  [unwired: 6 in]
        n193 = local write "SYS Status"("Set Real Power" ("Status")) -> ()
        n194 = Bundle("Modbus master out"=w808, "error out"=w807) -> (w806:T5)  [unwired: 1 in]
        n195 = Replace Array Subset(array=w812, new element=w806, index=w803) -> (w811:T3)
        n196 = Wait Until Next ms Multiple(millisecond multiple=u32 10) -> ()  [unwired: 1 out]
      }
      frame 15 {
        n197 = local read "SYS DER Index"() -> (w822:i32)
        n198 = local read "data"() -> (w821:T1)
        n199 = Index Array(array=w823, index=w822) -> (element=w832:T5)
        n200 = Unbundle By Name(w821) -> ("Variable 2 Setpoint"=w820:sgl)
        n201 = Type Cast(type=u32 0, x=w820) -> (*(type *) &x=w836:u32)
        n202 = Split Number(x=w836) -> (hi(x)=w834:u16, lo(x)=w833:u16)
        n203 = Unbundle(w832) -> ("Modbus master out"=w831:refnum<class "Modbus Master.lvclass">, "error out"=w830:errorcluster)
        n204 = Build Array(w834, w833) -> (w825:u16[])
        n205 = call-dynamic "Write Multiple Holding Registers.vi"("error in (no error)"=w830, "holding register values"=w825, "starting address"=u16 2038, "Modbus master in"=w831) -> ("error out"=w828:errorcluster, "Modbus master out"=w829:refnum<class "Modbus Master.lvclass">)  [unwired: 6 in]
        n206 = Bundle("Modbus master out"=w829, "error out"=w828) -> (w827:T5)  [unwired: 1 in]
        n207 = Replace Array Subset(array=w823, new element=w827, index=w822) -> (w824:T3)
        n208 = Wait Until Next ms Multiple(millisecond multiple=u32 50) -> ()  [unwired: 1 out]
      }
      frame 16 {
        # "V"
        n209 = local read "SYS DER Index"() -> (w841:i32)
        n210 = local read "data"() -> (w840:T1)
        n211 = Index Array(array=w843, index=w841) -> (element=w851:T5)
        n212 = Unbundle By Name(w840) -> ("Variable 1 Setpoint"=w839:sgl)
        n213 = Type Cast(type=u32 0, x=w839) -> (*(type *) &x=w855:u32)
        n214 = Split Number(x=w855) -> (hi(x)=w853:u16, lo(x)=w852:u16)
        n215 = Unbundle(w851) -> ("Modbus master out"=w850:refnum<class "Modbus Master.lvclass">, "error out"=w849:errorcluster)
        n216 = Build Array(w853, w852) -> (w844:u16[])
        n217 = call-dynamic "Write Multiple Holding Registers.vi"("error in (no error)"=w849, "holding register values"=w844, "starting address"=u16 2040, "Modbus master in"=w850) -> ("error out"=w847:errorcluster, "Modbus master out"=w848:refnum<class "Modbus Master.lvclass">)  [unwired: 6 in]
        n218 = Bundle("Modbus master out"=w848, "error out"=w847) -> (w846:T5)  [unwired: 1 in]
        n219 = Replace Array Subset(array=w843, new element=w846, index=w841) -> (w842:T3)
        n220 = Wait Until Next ms Multiple(millisecond multiple=u32 50) -> ()  [unwired: 1 out]
      }
      frame 17 {
        n221 = local read "SYS DER Index"() -> (w860:i32)
        n222 = local read "data"() -> (w859:T1)
        n223 = Index Array(array=w862, index=w860) -> (element=w870:T5)
        n224 = Unbundle By Name(w859) -> ("Variable 2 Setpoint"=w858:sgl)
        n225 = Type Cast(type=u32 0, x=w858) -> (*(type *) &x=w874:u32)
        n226 = Split Number(x=w874) -> (hi(x)=w872:u16, lo(x)=w871:u16)
        n227 = Unbundle(w870) -> ("Modbus master out"=w869:refnum<class "Modbus Master.lvclass">, "error out"=w868:errorcluster)
        n228 = Build Array(w872, w871) -> (w863:u16[])
        n229 = call-dynamic "Write Multiple Holding Registers.vi"("error in (no error)"=w868, "holding register values"=w863, "starting address"=u16 2042, "Modbus master in"=w869) -> ("error out"=w866:errorcluster, "Modbus master out"=w867:refnum<class "Modbus Master.lvclass">)  [unwired: 6 in]
        n230 = Bundle("Modbus master out"=w867, "error out"=w866) -> (w865:T5)  [unwired: 1 in]
        n231 = Replace Array Subset(array=w862, new element=w865, index=w860) -> (w861:T3)
        n232 = Wait Until Next ms Multiple(millisecond multiple=u32 250) -> ()  [unwired: 1 out]
      }
      frame 1000 {
        n233 = property class="VI"(reference=w878) -> ("Exec.State"=w879:T6)  [unwired: 1 in, 2 out]
        n234 = case shown="\"Idle\"" w879 {
          tunnel: w880 -> [_ w894 _ _]
          tunnel: w878 -> [_ w884 w903 w905]
          tunnel: [0 0 1000 1000] -> w877
          frame "Bad", Default {
          }
          frame "Idle" {
            n235 = invoke class="VI" method="Run VI"(reference=w884, "Wait until done"=FALSE ("Wait Until Done"), "Auto Dispose Ref"=FALSE ("Auto Dispose Reference")) -> (reference out=w890:refnum<vi>)  [unwired: 2 in, 4 out]
            n236 = local read "SYS DER Index"() -> (w897:i32)
            n237 = invoke class="VI" method="FP.Open"(reference=w890, "Activate"=TRUE ("Activate?"), "State"=T4."Standard") -> (reference out=w889:refnum<vi>)  [unwired: 2 in, 4 out]
            n238 = To Variant(anything=w897) -> (Variant=w899:variant)
            n239 = invoke class="VI" method="Ctrl Val.Set"(reference=w889, "Control Name"="DER", "Value"=w899) -> (reference out=w895:refnum<vi>)  [unwired: 2 in, 4 out]
            n240 = To Variant(anything=w894) -> (Variant=w896:variant)
            n241 = invoke class="VI" method="Ctrl Val.Set"(reference=w895, "Control Name"="Event", "Value"=w896) -> (reference out=w886:refnum<vi>)  [unwired: 2 in, 4 out]
            n242 = To Variant(anything="DER List") -> (Variant=w888:variant)
            n243 = invoke class="VI" method="Ctrl Val.Set"(reference=w886, "Control Name"="DER Names", "Value"=w888) -> ()  [unwired: 2 in, 5 out]
          }
          frame "Run top level" {
            n244 = invoke class="VI" method="Abort VI"(reference=w903) -> ()  [unwired: 2 in, 3 out]
          }
          frame "Running" {
            n245 = invoke class="VI" method="Abort VI"(reference=w905) -> ()  [unwired: 2 in, 3 out]
          }
        }
      }
      frame 1001 {
        n246 = property class="VI"(reference=w906) -> ("Exec.State"=w908:T6)  [unwired: 1 in, 2 out]
        n247 = case shown="\"Idle\"" w908 {
          tunnel: w906 -> [_ w917 w927 w929]
          tunnel: [0 0 1000 1000] -> w907
          frame "Bad", Default {
          }
          frame "Idle" {
            n248 = invoke class="VI" method="Run VI"(reference=w917, "Wait until done"=FALSE ("Wait Until Done"), "Auto Dispose Ref"=FALSE ("Auto Dispose Reference")) -> (reference out=w913:refnum<vi>)  [unwired: 2 in, 4 out]
            n249 = local read "SYS DER Index"() -> (w923:i32)
            n250 = invoke class="VI" method="FP.Open"(reference=w913, "Activate"=TRUE ("Activate?"), "State"=T4."Standard") -> (reference out=w914:refnum<vi>)  [unwired: 2 in, 4 out]
            n251 = To Variant(anything=w923) -> (Variant=w925:variant)
            n252 = invoke class="VI" method="Ctrl Val.Set"(reference=w914, "Control Name"="DER", "Value"=w925) -> (reference out=w918:refnum<vi>)  [unwired: 2 in, 4 out]
            n253 = local read "DER List"() -> (w919:string[])
            n254 = To Variant(anything=w919) -> (Variant=w921:variant)
            n255 = invoke class="VI" method="Ctrl Val.Set"(reference=w918, "Control Name"="DER Names", "Value"=w921) -> ()  [unwired: 2 in, 5 out]
          }
          frame "Run top level" {
            n256 = invoke class="VI" method="Abort VI"(reference=w927) -> ()  [unwired: 2 in, 3 out]
          }
          frame "Running" {
            n257 = invoke class="VI" method="Abort VI"(reference=w929) -> ()  [unwired: 2 in, 3 out]
          }
        }
      }
    }
    n258 = local read "ALL Real Power"() -> (w107:sgl[])
    n259 = for {
      tunnel: w107 -> [w123] mode=indexing
      i -> [w128]
      n260 = Greater?(x=w123, y=sgl 200.0) -> (0:w136:bool)
      n261 = Less?(x=w123, y=sgl -200.0) -> (x < y?=w135:bool)
      n262 = Greater?(x=w123, y=sgl 1000.0) -> (0:w122:bool)
      n263 = Less?(x=w123, y=sgl -1000.0) -> (x < y?=w121:bool)
      n264 = Greater?(x=w123, y=sgl 5000.0) -> (0:w120:bool)
      n265 = Less?(x=w123, y=sgl -5000.0) -> (x < y?=w119:bool)
      n266 = Build Array(w136, w135, w122, w121, w120, w119) -> (w134:bool[])
      n267 = local read "SYS Iteration"() -> (w130:i32)
      n268 = Boolean Array To Number(Boolean array=w134) -> (number=w132:u32)
      n269 = Quotient & Remainder(x=w130, y=3) -> (x-y*floor(x/y)=w129:i32)  [unwired: 1 out]
      n270 = case shown="42" w132 {
        tunnel: [0 ("x") w143 w169 w196 w223 w251 w279] -> w133
        tunnel: w129 -> [_ w141 w168 w194 w221 w249 w277]
        tunnel: w128 -> [_ w140 w166 w197 w225 w253 w281]
        frame 0, Default {
        }
        frame 1 {
          # "> 500W"
          n271 = case shown="4" w140 {
            tunnel: [1 ("x") 1 ("x") 4 ("x") 1 ("x") 1 ("x") 4 ("x") 1 ("x") 4 ("x") 1 ("x") 4 ("x") 1 ("x") 4 ("x") 1 ("x") 4 ("x") 1 ("x") 1 ("x") 4 ("x") 4 ("x") 1 ("x") 1 ("x") 1 ("x") 1 ("x")] -> w142
            frame 0, Default {
            }
            frame 1 {
            }
            frame 2 {
            }
            frame 3 {
            }
            frame 4 {
            }
            frame 5 {
            }
            frame 6 {
            }
            frame 7 {
            }
            frame 8 {
            }
            frame 9 {
            }
            frame 10 {
            }
            frame 11 {
            }
            frame 12 {
            }
            frame 13 {
            }
            frame 14 {
            }
            frame 15 {
            }
            frame 16 {
            }
            frame 17 {
            }
            frame 18 {
            }
            frame 19 {
            }
            frame 20 {
            }
            frame 21 {
            }
          }
          n272 = Add(x=w142, y=w141) -> (x+y=w143:i32)
        }
        frame 2 {
          # "< -500W"
          n273 = case shown="4" w166 {
            tunnel: [4 ("x") 4 ("x") 1 ("x") 4 ("x") 4 ("x") 1 ("x") 4 ("x") 1 ("x") 4 ("x") 1 ("x") 4 ("x") 1 ("x") 4 ("x") 1 ("x") 4 ("x") 4 ("x") 1 ("x") 1 ("x") 4 ("x") 4 ("x") 4 ("x") 4 ("x")] -> w167
            frame 0, Default {
            }
            frame 1 {
            }
            frame 2 {
            }
            frame 3 {
            }
            frame 4 {
            }
            frame 5 {
            }
            frame 6 {
            }
            frame 7 {
            }
            frame 8 {
            }
            frame 9 {
            }
            frame 10 {
            }
            frame 11 {
            }
            frame 12 {
            }
            frame 13 {
            }
            frame 14 {
            }
            frame 15 {
            }
            frame 16 {
            }
            frame 17 {
            }
            frame 18 {
            }
            frame 19 {
            }
            frame 20 {
            }
            frame 21 {
            }
          }
          n274 = Add(x=w167, y=w168) -> (x+y=w169:i32)
        }
        frame 5 {
          # "> 2000W"
          n275 = case shown="4" w197 {
            tunnel: [1 ("x") 1 ("x") 4 ("x") 1 ("x") 1 ("x") 4 ("x") 1 ("x") 4 ("x") 1 ("x") 4 ("x") 1 ("x") 4 ("x") 1 ("x") 4 ("x") 1 ("x") 1 ("x") 4 ("x") 4 ("x") 1 ("x") 1 ("x") 1 ("x") 1 ("x")] -> w195
            frame 0, Default {
            }
            frame 1 {
            }
            frame 2 {
            }
            frame 3 {
            }
            frame 4 {
            }
            frame 5 {
            }
            frame 6 {
            }
            frame 7 {
            }
            frame 8 {
            }
            frame 9 {
            }
            frame 10 {
            }
            frame 11 {
            }
            frame 12 {
            }
            frame 13 {
            }
            frame 14 {
            }
            frame 15 {
            }
            frame 16 {
            }
            frame 17 {
            }
            frame 18 {
            }
            frame 19 {
            }
            frame 20 {
            }
            frame 21 {
            }
          }
          n276 = Add(x=6, y=w194) -> (x+y=w192:i32)
          n277 = Add(x=w195, y=w192) -> (x+y=w196:i32)
        }
        frame 10 {
          # "< -2000W"
          n278 = case shown="12" w225 {
            tunnel: [4 ("x") 4 ("x") 1 ("x") 4 ("x") 4 ("x") 1 ("x") 4 ("x") 1 ("x") 4 ("x") 1 ("x") 4 ("x") 1 ("x") 4 ("x") 1 ("x") 4 ("x") 4 ("x") 1 ("x") 1 ("x") 4 ("x") 4 ("x") 4 ("x") 4 ("x")] -> w224
            frame 0, Default {
            }
            frame 1 {
            }
            frame 2 {
            }
            frame 3 {
            }
            frame 4 {
            }
            frame 5 {
            }
            frame 6 {
            }
            frame 7 {
            }
            frame 8 {
            }
            frame 9 {
            }
            frame 10 {
            }
            frame 11 {
            }
            frame 12 {
            }
            frame 13 {
            }
            frame 14 {
            }
            frame 15 {
            }
            frame 16 {
            }
            frame 17 {
            }
            frame 18 {
            }
            frame 19 {
            }
            frame 20 {
            }
            frame 21 {
            }
          }
          n279 = Add(x=6, y=w221) -> (x+y=w220:i32)
          n280 = Add(x=w224, y=w220) -> (x+y=w223:i32)
        }
        frame 21 {
          # "> 8000W"
          n281 = case shown="12" w253 {
            tunnel: [1 ("x") 1 ("x") 4 ("x") 1 ("x") 1 ("x") 4 ("x") 1 ("x") 4 ("x") 1 ("x") 4 ("x") 1 ("x") 4 ("x") 1 ("x") 4 ("x") 1 ("x") 1 ("x") 4 ("x") 4 ("x") 1 ("x") 1 ("x") 1 ("x") 1 ("x")] -> w252
            frame 0, Default {
            }
            frame 1 {
            }
            frame 2 {
            }
            frame 3 {
            }
            frame 4 {
            }
            frame 5 {
            }
            frame 6 {
            }
            frame 7 {
            }
            frame 8 {
            }
            frame 9 {
            }
            frame 10 {
            }
            frame 11 {
            }
            frame 12 {
            }
            frame 13 {
            }
            frame 14 {
            }
            frame 15 {
            }
            frame 16 {
            }
            frame 17 {
            }
            frame 18 {
            }
            frame 19 {
            }
            frame 20 {
            }
            frame 21 {
            }
          }
          n282 = Add(x=12, y=w249) -> (x+y=w248:i32)
          n283 = Add(x=w252, y=w248) -> (x+y=w251:i32)
        }
        frame 42 {
          # "< -8000W"
          n284 = case shown="12" w281 {
            tunnel: [4 ("x") 4 ("x") 1 ("x") 4 ("x") 4 ("x") 1 ("x") 4 ("x") 1 ("x") 4 ("x") 1 ("x") 4 ("x") 1 ("x") 4 ("x") 1 ("x") 4 ("x") 4 ("x") 1 ("x") 1 ("x") 4 ("x") 4 ("x") 4 ("x") 4 ("x")] -> w280
            frame 0, Default {
            }
            frame 1 {
            }
            frame 2 {
            }
            frame 3 {
            }
            frame 4 {
            }
            frame 5 {
            }
            frame 6 {
            }
            frame 7 {
            }
            frame 8 {
            }
            frame 9 {
            }
            frame 10 {
            }
            frame 11 {
            }
            frame 12 {
            }
            frame 13 {
            }
            frame 14 {
            }
            frame 15 {
            }
            frame 16 {
            }
            frame 17 {
            }
            frame 18 {
            }
            frame 19 {
            }
            frame 20 {
            }
            frame 21 {
            }
          }
          n285 = Add(x=12, y=w277) -> (x+y=w276:i32)
          n286 = Add(x=w280, y=w276) -> (x+y=w279:i32)
        }
      }
      n287 = case shown="1" w128 {
        tunnel: w133 -> [w304 w305 w306 w307 w308 w309 w310 w311 w312 w313 w314 w315 w316]
        frame 0, Default {
          "DER0 Flow" <- w304
        }
        frame 1 {
          "DER1 Flow" <- w305
        }
        frame 2 {
          "DER2 Flow" <- w306
        }
        frame 3 {
          "DER3 Flow" <- w307
        }
        frame 4 {
          "DER4 Flow" <- w308
        }
        frame 5 {
          "DER5 Flow" <- w309
        }
        frame 6 {
          "DER6 Flow" <- w310
        }
        frame 7 {
          "DER7 Flow" <- w311
        }
        frame 8 {
          "DER8 Flow" <- w312
        }
        frame 9 {
          "DER9 Flow" <- w313
        }
        frame 10 {
          "DER10 Flow" <- w314
        }
        frame 11 {
          "DER11 Flow" <- w315
        }
        frame 12 {
          "DER12 Flow" <- w316
        }
      }
    }
    n288 = local write "SYS Case"(w82) -> ()
    n289 = for {
      tunnel: w111 -> [w319] mode=indexing
      tunnel: [w318] -> w110 mode=indexing
      tunnel: [w319] -> w108 mode=indexing
      tunnel: [w317] -> w109 mode=indexing
      n290 = Unbundle(w319) -> ("error out"=w318:errorcluster)  [unwired: 1 out]
      n291 = Unbundle By Name(w318) -> ("status"=w317:bool)
    }
    "ALL DER Current Error" <- w110
    "ALL Error Indicator" <- w109
  }
  n292 = Close File(refnum=w22, error in=w21) -> (error out=→"error out 3":errorcluster)  [unwired: 1 out]
  n293 = for {
    tunnel: w27 -> [w933] mode=indexing
    tunnel: [w930] -> w31 mode=indexing
    n294 = Unbundle(w933) -> ("Modbus master out"=w932:refnum<class "Modbus Master.lvclass">, "error out"=w931:errorcluster)
    n295 = call-dynamic "Close.vi"("error in (no error)"=w931, "Modbus master in"=w932) -> ("error out"=w930:errorcluster)  [unwired: 9 in]
  }
  "ALL DER Final Error" <- w31
  n296 = Unregister For Events(event registration refnum=w9) -> ()  [unwired: 1 in, 1 out]
  n297 = Destroy User Event(user event=w8) -> ()  [unwired: 1 in, 1 out]
  n298 = Destroy User Event(user event=w5) -> ()  [unwired: 1 in, 1 out]
  "SYS Iteration" <- 0
  "SYS DER Index" <- 0 ("DER Index")
  "SYS Status" <- "Initializing" ("Sys Status")
  "SYS Case" <- 0 ("SYS Case")
